vi "tcpSysTxFreqFromZ.vi"(8 "error in (no error)":errorcluster, 9 "timeout (ms)":i32=40000, 10 "txFrequencyHz in":sgl, 11 "connection ID in":refnum<k5>) -> (0 "error out":errorcluster, 1 "TxFreqIndex":i8, 2 "txFrequencyHz out":sgl=1000000.0, 3 "connection ID out":refnum<k5>, 5 "SysTxFreqHzA":sgl[](array[numeric])=[1000000.0, 1111100.0, 1250000.0, 1333300.0, 1428600.0, 1538500.0, 1666700.0, 1818200.0, 2000000.0, 2222200.0, 2500000.0, 2666700.0, 2857100.0, 3076900.0, 3333300.0, 3636400.0, 3809500.0, 4000000.0, 4210500.0, 4444400.0, 4705900.0, 5000000.0, 5333300.0, 5714300.0, 6153800.0, 6666700.0, 7272700.0, 8000000.0, 8888900.0, 10000000.0, 11428600.0])   [LabVIEW 2016]
doc: "Reads all allowed transmit frequencies from the Z system, and finds the one closest to the input frequency. It creates an array of commands to read frequencies from:\n Hardware Control Layer.\n Beamforming.\n Common.\n SysTxFreqHzA\nand sends them using tcpCmdArrayToZ. It returns an array of all frequencies, and the index and value of the one closest to the input frequency."
uses:
  TemperatureMeasure/Thermal_type.vi
panel:
  # "Program constants"
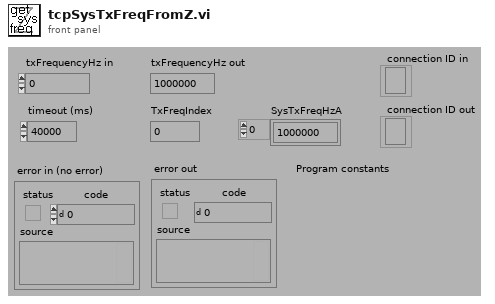
[diagram p1: front panel]
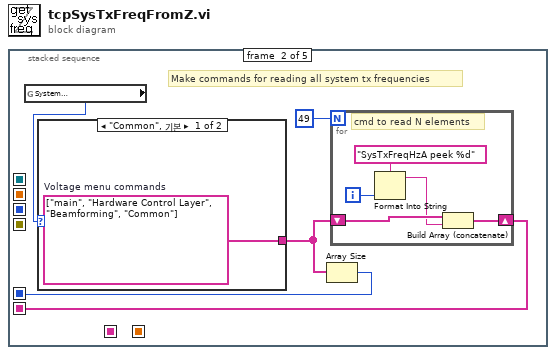
[diagram p0: block diagram]
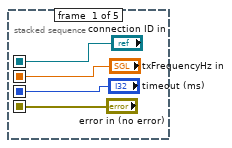
[diagram p2: hidden frame]
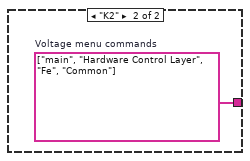
[diagram p3: hidden frame]
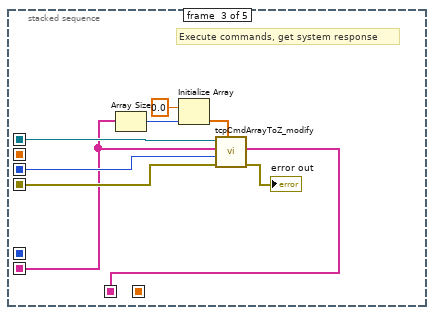
[diagram p4: hidden frame]
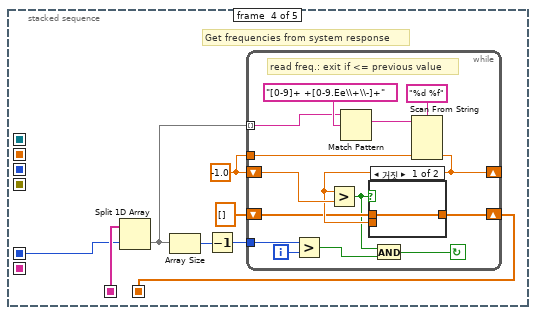
[diagram p5: hidden frame]
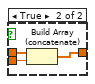
[diagram p6: hidden frame]
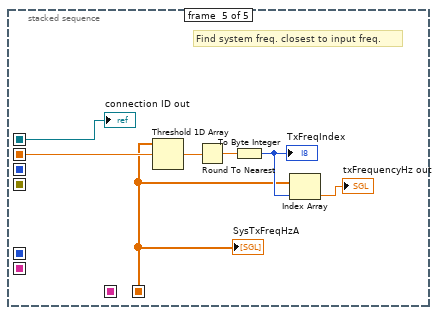
[diagram p7: hidden frame]
diagram:
  n1 = stacked-sequence {
    seq-local: ["connection ID in" _ _ _ _] -> [_ _ w25 _ w53]
    seq-local: ["txFrequencyHz in" _ _ _ _] -> [_ _ _ _ w58]
    seq-local: ["error in (no error)" _ _ _ _] -> [_ _ w24 _ _]
    seq-local: [_ w9 _ _ _] -> [_ _ w21 _ _]
    seq-local: ["timeout (ms)" _ _ _ _] -> [_ _ w23 _ _]
    seq-local: [_ w7 _ _ _] -> [_ _ _ w28 _]
    seq-local: [_ _ _ w26 _] -> [_ _ _ _ w52]
    seq-local: [_ _ w17 _ _] -> [_ _ _ w29 _]
    frame #0 {
    }
    frame #1 {
      # "Make commands for reading all system tx frequencies"
      n2 = global read "Thermal_type.vi" "System \nSelection"() -> (w6:enum32{"Common", "Frosk", "Griffin", "K2"})
      n3 = case shown="\"Common\", 기본" w6 {
        tunnel: [w10 w11] -> w5
        frame "Common", Default {
          w10 = string[] ["main", "Hardware Control Layer", "Beamforming", "Common"]  # Voltage menu commands
        }
        frame "K2" {
          w11 = string[] ["main", "Hardware Control Layer", "Fe", "Common"]  # Voltage menu commands
        }
      }
      n4 = Array Size(array=w5) -> (size(s)=w7:i32)
      n5 = for {
        N: 49 -> [_]
        shift-right: [w12] -> w9
        shift-left: w5 -> [w14]
        i -> [w15]
        # "cmd to read N elements"
        n6 = Format Into String(format string="SysTxFreqHzA peek %d" ("Format String"), w15) -> (resulting string=w13:string)  [unwired: 2 in, 1 out]
        n7 = Build Array (concatenate)(w14, w13) -> (w12:string[])
      }
    }
    frame #2 {
      # "Execute commands, get system response"
      n8 = Array Size(array=w21) -> (size(s)=w20:i32)
      n9 = Initialize Array(sgl 0.0 ("Element Data"), w20) -> (w19:sgl[])
      n10 = call "tcpCmdArrayToZ_modify.vi"("Delay (sec)"=w19, "error in (no error)"=w24, "Timeout (ms)"=w23, "Command array"=w21, "connection ID in"=w25) -> ("error out"=→"error out":errorcluster, "Receive array"=w17:string[])  [unwired: 2 in, 3 out]
    }
    frame #3 {
      w33 = sgl -1.0 ("Default Value 2")
      # "Get frequencies from system response"
      n11 = Split 1D Array(array=w29, index=w28) -> (second subarray=w27:string[])  [unwired: 1 out]
      n12 = Array Size(array=w27) -> (size(s)=w31:i32)
      n13 = Decrement(x=w31) -> (x-1=w30:i32)
      n14 = while {
        tunnel: w30 -> [w38]
        tunnel: w33 -> [w43]
        shift-left: sgl[] [] ("Array Constant") -> [w40]
        shift-right: [w39] -> w26
        shift-left: w33 -> [w42]
        shift-right: [w41] -> _
        tunnel: w27 -> [w44] mode=indexing
        i -> [w37]
        stop <- w34 continue-if-true
        # "read freq.: exit if <= previous value"
        n15 = Greater?(x=w38, y=w37) -> (0:w35:bool)
        n16 = Match Pattern(string=w44, regular expression="[0-9]+ +[0-9.Ee\\+\\-]+") -> (match substring=w46:string)  [unwired: 1 in, 3 out]
        n17 = Scan From String(format string="%d %f" ("Format String"), input string=w46, default 2=w43) -> (output 2=w41:sgl)  [unwired: 4 in, 3 out]
        n18 = Greater?(x=w41, y=w42) -> (0:w36:bool)
        n19 = case shown="거짓" w36 {
          tunnel: w41 -> [_ w51]
          tunnel: w40 -> [w48 w50]
          tunnel: [w48 w49] -> w39
          frame False {
          }
          frame True {
            n20 = Build Array (concatenate)(w50, w51) -> (w49:sgl[])
          }
        }
        n21 = And(x=w36, y=w35) -> (x .and. y?=w34:bool)
      }
    }
    frame #4 {
      # "Find system freq. closest to input freq."
      n22 = Threshold 1D Array(2:w58, 3:w52) -> (0:w57:sgl)  [unwired: 1 in]
      n23 = Round To Nearest(number=w57) -> (nearest integer value=w56:sgl)
      n24 = To Byte Integer(number=w56) -> (8bit integer=w55:i8)
      "TxFreqIndex" <- w55
      n25 = Index Array(array=w52, index=w55) -> (element=→"txFrequencyHz out":sgl)
      "SysTxFreqHzA" <- w52
      "connection ID out" <- w53
    }
  }
